vi "檔案_Offset.vi"() -> ()   [LabVIEW 2015]
panel:
  out "存檔":bool
  in  "Save Button":bool
  out "Recipe Ring":string
  in  "Exit":bool
  # "Recipe - 各工站微調表(mm)"
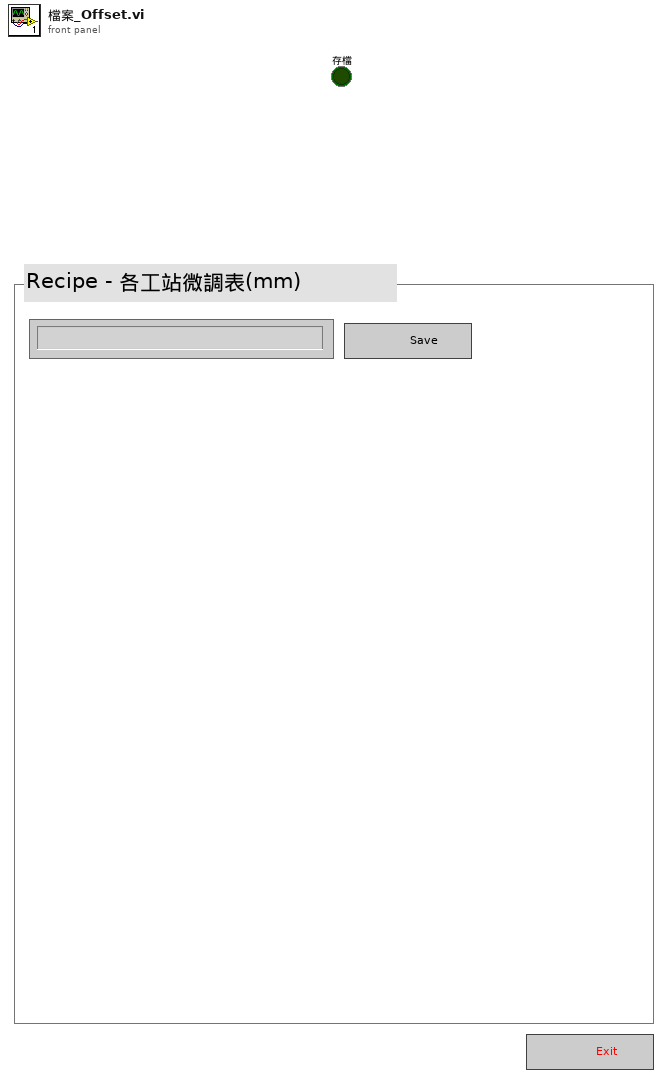
[diagram p1: front panel]
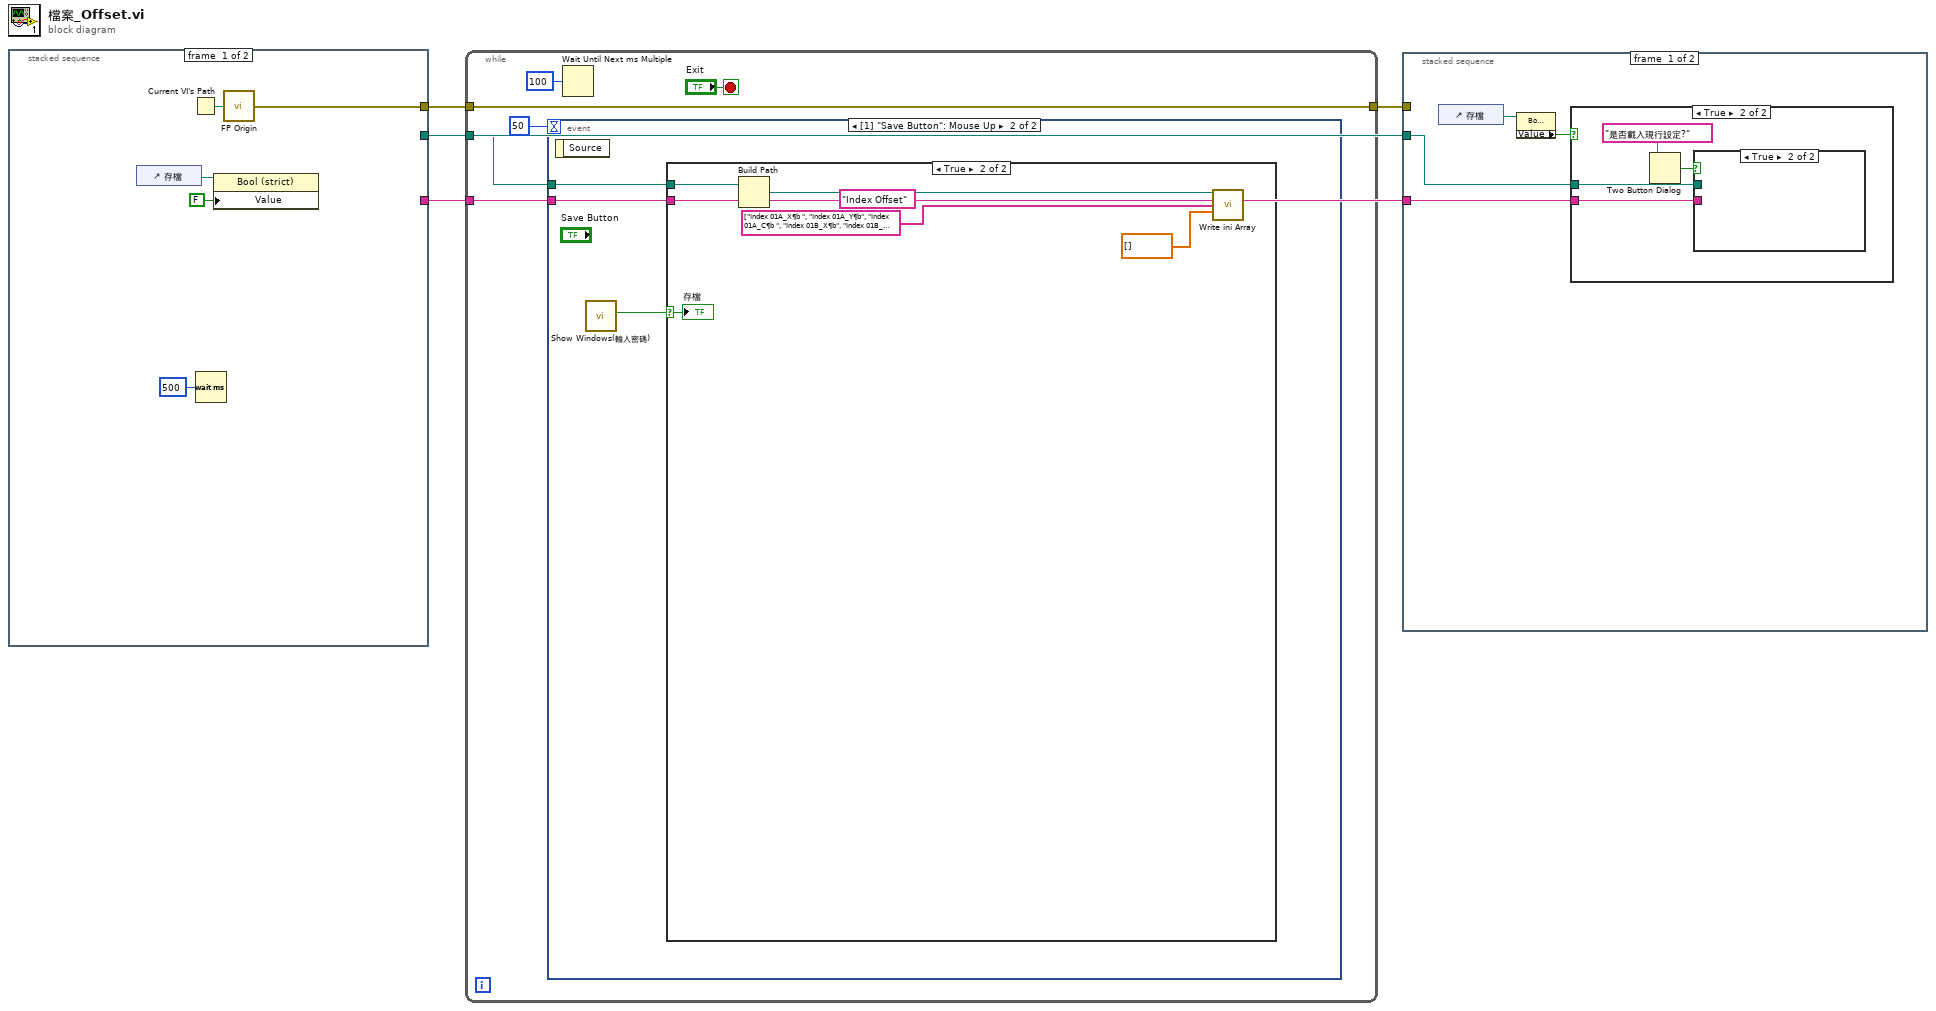
[diagram p0: block diagram]
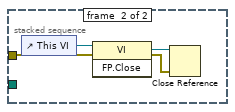
[diagram p4: hidden frame]
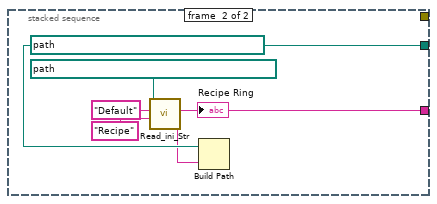
[diagram p5: hidden frame]
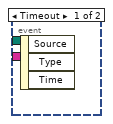
[diagram p6: hidden frame]
diagram:
  n1 = stacked-sequence {
    tunnel: [w8 _] -> w3
    tunnel: [_ w10] -> w1
    tunnel: [_ w11] -> w2
    frame #0 {
      n2 = control-ref of="存檔"() -> (w6:refnum<vi>)
      n3 = Current VI's Path() -> (path=w9:path)
      n4 = Wait (ms)(milliseconds to wait=u32 500) -> ()  [unwired: 1 out]
      n5 = property class="Bool (strict)"(reference=w6, "Value"=FALSE) -> ()  [unwired: 1 in, 2 out]
      n6 = call "FP Origin.vi"("vi path"=w9) -> ("error out"=w8:errorcluster)
    }
    frame #1 {
      w11 = path "D:/Folding自動機 Data/Recipe/Position" ("configuration file path")
      n7 = call "Read_ini_Str.vi"("key"="Recipe", "section"="Default", "configuration file path"=path "D:/Folding自動機 Data/Recipe/Default.ini") -> ("value"=w10:string)  [unwired: 7 in, 1 out]
      "Recipe Ring" <- w10
      n8 = Build Path(base path=w11, name or relative path=w10) -> ()  [unwired: 1 out]
    }
  }
  n9 = while {
    tunnel: w3 -> [w17]
    tunnel: [w17] -> w4
    tunnel: w1 -> [w16]
    tunnel: w2 -> [w15]
    stop <- "Exit" stop-if-true
    n10 = event shown="[1] \"Save Button\": Mouse Up" {
      selector: _ -> [_ _]
      dyn-events: _ -> [_ _]
      timeout: 50 -> [_ _]
      tunnel: w16 -> [_ w23]
      tunnel: w15 -> [_ w22]
      event Timeout {
        n11 = event-data() -> ()  [unwired: 1 in, 3 out]
      }
      event "Save Button": Mouse Up {
        n12 = event-data() -> ()  [unwired: 1 in, 1 out]
        n13 = call "Show Windows(輸入密碼).vi"() -> ("密碼正確"=w21:bool)  [unwired: 10 in, 1 out]
        n14 = case shown="True" w21 {
          selector: w21 -> [_ w25]
          tunnel: w23 -> [_ w30]
          tunnel: w22 -> [_ w29]
          frame False {
          }
          frame True {
            n15 = Build Path(base path=w29, name or relative path=w30) -> (appended path=w28:path)
            n16 = call "Write ini Array.vi"("configuration file path"=w28, "section"="Index Offset" ("key"), "KeysArray"=string[] ["Index 01A_X¶b ", "Index 01A_Y¶b", "Index 01A_C¶b ", "Index 01B_X¶b", "Index 01B_Y¶b", "Index 01B_C¶b", "Index 02A_X¶b", "Index 02A_Y¶b", "Index 02A_C¶b", "Index 02B_X¶b", "Index 02B_Y¶b", "Index 02B_C¶b", "Index 03A_X¶b", "Index 03A_Y¶b", "Index 03A_C¶b", "Index 03B_X¶b", "Index 03B_Y¶b", "Index 03B_C¶b", "Index 04A_X¶b", "Index 04A_Y¶b", "Index 04A_C¶b", "Index 04B_X¶b", "Index 04B_Y¶b", "Index 04B_C¶b", "Index 05A_X¶b", "Index 05A_Y¶b", "Index 05A_C¶b", "Index 05B_X¶b", "Index 05B_Y¶b", "Index 05B_C¶b", "Index 06A_X¶b", "Index 06A_Y¶b", "Index 06A_C¶b", "Index 06B_X¶b", "Index 06B_Y¶b", "Index 06B_C¶b", "Index 07A_X¶b", "Index 07A_Y¶b", "Index 07A_C¶b", "Index 07B_X¶b", "Index 07B_Y¶b", "Index 07B_C¶b", "Index 08A_X¶b", "Index 08A_Y¶b", "Index 08A_C¶b", "Index 08B_X¶b", "Index 08B_Y¶b", "Index 08B_C¶b"], "ValueArray"=dbl[] []) -> ()  [unwired: 11 in, 1 out]
            "存檔" <- w25
          }
        }
      }
    }
    n17 = Wait Until Next ms Multiple(millisecond multiple=u32 100) -> ()  [unwired: 1 out]
  }
  n18 = stacked-sequence {
    tunnel: w4 -> [_ w42]
    tunnel: w2 -> [w34 _]
    tunnel: w1 -> [w33 _]
    frame #0 {
      n19 = control-ref of="存檔"() -> (w32:refnum<vi>)
      n20 = property class="Bool (strict)"(reference=w32) -> ("Value"=w31:bool)  [unwired: 1 in, 2 out]
      n21 = case shown="True" w31 {
        tunnel: w34 -> [_ w36]
        tunnel: w33 -> [_ w35]
        frame False {
        }
        frame True {
          n22 = Two Button Dialog(message="是否載入現行設定?") -> (T button?=w38:bool)  [unwired: 2 in]
          n23 = case shown="True" w38 {
            tunnel: w36 -> [_ _]
            tunnel: w35 -> [_ _]
            frame False {
            }
            frame True {
            }
          }
        }
      }
    }
    frame #1 {
      n24 = control-ref of="This VI"() -> (w41:refnum<vi>)
      n25 = invoke class="VI" method="FP.Close"(reference=w41, error in=w42) -> (reference out=w40:refnum<vi>, error out=w39:errorcluster)  [unwired: 1 in, 1 out]
      n26 = Close Reference(reference=w40, error in (no error)=w39) -> ()  [unwired: 1 out]
    }
  }
